vi "Server Cmd Answer - Get Status.vi"(7 "server event ref":refnum<vi>, 8 "error in":errorcluster, 10 "message":string, 11 "Status ready? (False)":bool) -> (0 "error out":errorcluster, 3 "info data out":string)   [LabVIEW 2018]
doc: "Send answer for command \"Get status\"."
uses:
  octave/infolib.lvlibp/Private/Add key polymorph parts/String.vi
  octave/infolib.lvlibp
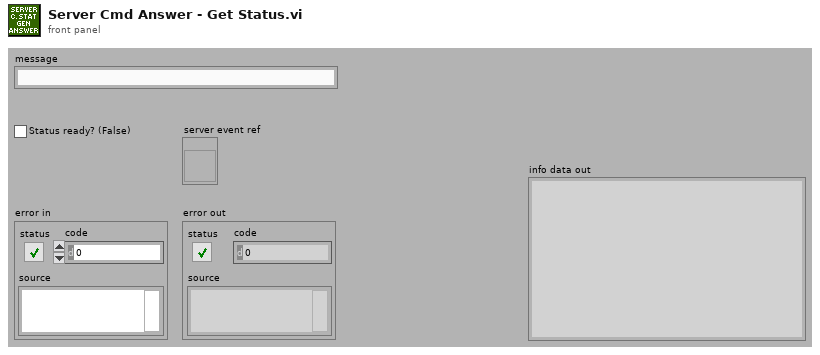
[diagram p1: front panel]
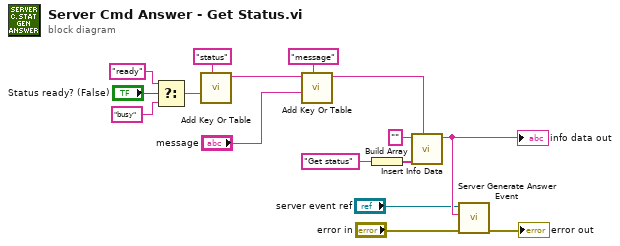
[diagram p0: block diagram]
diagram:
  n1 = Select(t="ready" ("string"), s="Status ready? (False)", f="busy" ("string")) -> (s? t:f=w1:string)
  n2 = call-poly "Add Key Or Table.vi"("key description"="status", "string"=w1) -> ("info data out"=w14:string)  [unwired: 8 in, 1 out]
  n3 = call-poly "Add Key Or Table.vi"("key description"="message", "string"="message", "info data"=w14) -> ("info data out"=w13:string)  [unwired: 7 in, 1 out]
  n4 = Build Array("Get status" ("key description")) -> (w12:string[])
  n5 = call "Insert Info Data.vi"("info data to insert"=w13, "sections"=w12, "info data"="") -> ("info data out"=w10:string)  [unwired: 7 in, 1 out]
  "info data out" <- w10
  n6 = call "Server Generate Answer Event.vi"("error in"="error in", "event data"=w10, "server event ref"="server event ref") -> ("error out"=→"error out":errorcluster)  [unwired: 8 in]
